vi "getTraceScreen.vi"(8 "error in":errorcluster, 11 "VISA in":refnum<visa-resource-name>="TCPIP0::172.16.1.100::inst0::INSTR") -> (0 "error out":errorcluster, 3 "VISA out":refnum<visa-resource-name>)   [LabVIEW 2023, in "Keysight.lvlib"]
uses:
  Keysight.lvlib
panel:
  out "*OPC?":string
  in  "FileName":string="FileName"
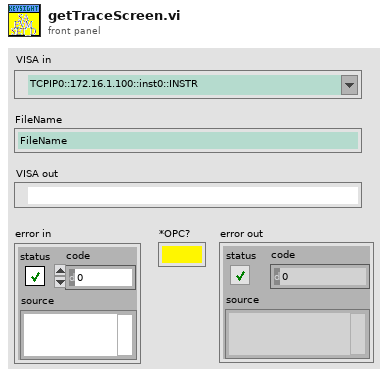
[diagram p1: front panel]
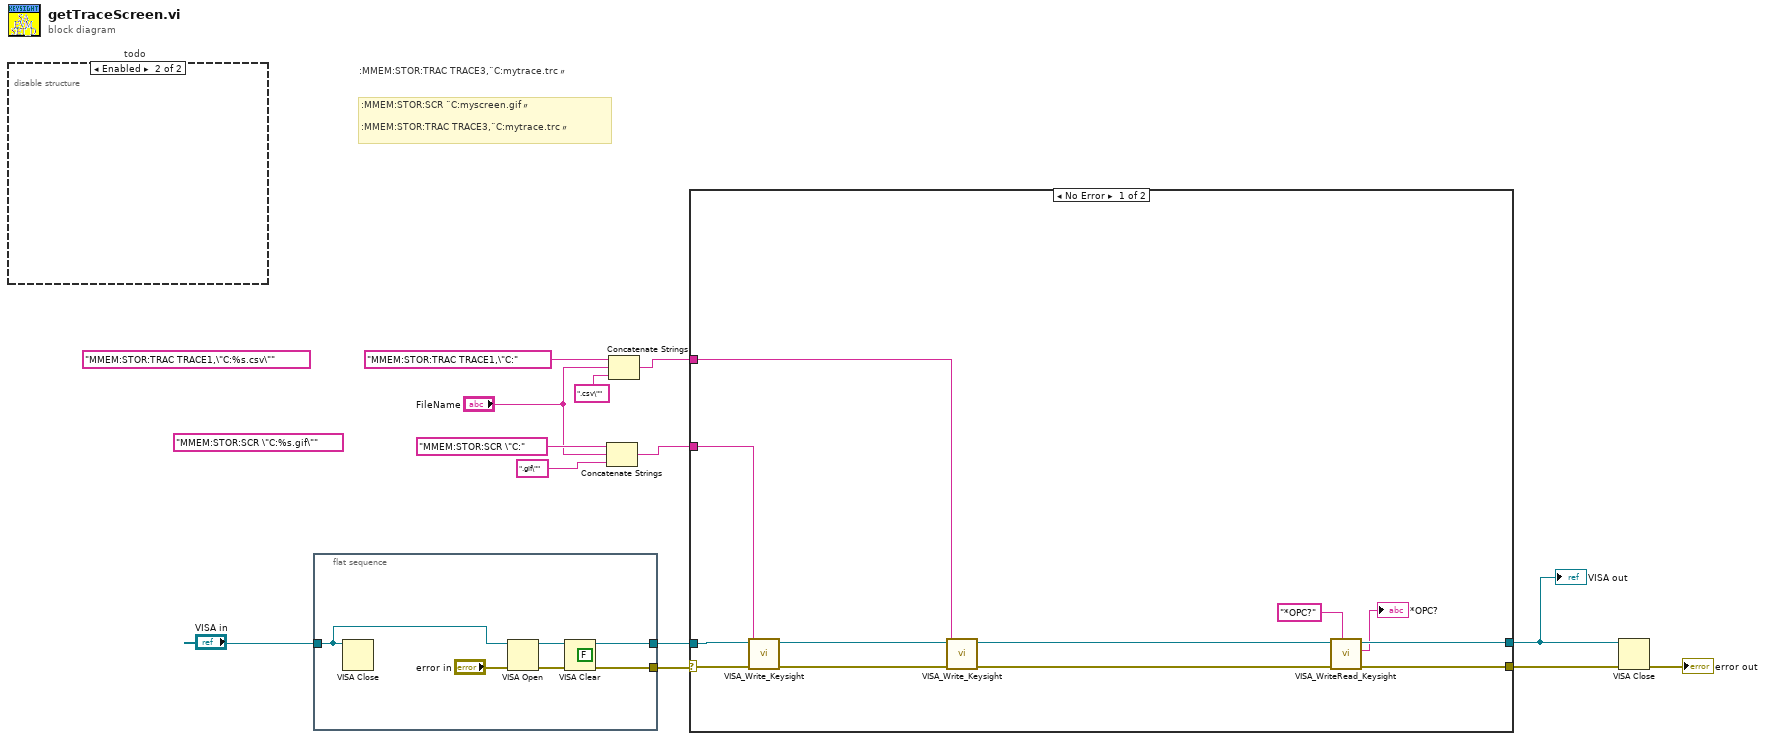
[diagram p0: block diagram]
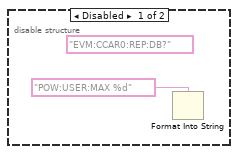
[diagram p2: hidden frame]
diagram:
  (unwired) "MMEM:STOR:TRAC TRACE1,\"C:%s.csv\"" ("write buffer")
  (unwired) "MMEM:STOR:SCR \"C:%s.gif\"" ("write buffer")
  # ":MMEM:STOR:SCR ¨C:myscreen.gif〃\n\n:MMEM:STOR:TRAC TRACE3,¨C:mytrace.trc〃"
  # ":MMEM:STOR:TRAC TRACE3,¨C:mytrace.trc〃"
  n1 = disable-structure "todo" shown="Enabled" {
    frame Disabled {
      (unwired) "EVM:CCAR0:REP:DB?" ("write buffer")
      n2 = Format Into String(format string="POW:USER:MAX %d") -> ()  [unwired: 3 in, 2 out]
    }
    frame Enabled {
    }
  }
  n3 = flat-sequence {
    tunnel: [w18] -> w6
    tunnel: [w17] -> w5
    tunnel: "VISA in" -> [w16]
    frame #0 {
      (unwired) FALSE ("duplicate session (F)")
      n4 = VISA Close(VISA resource name=w16) -> ()  [unwired: 1 in, 1 out]
      n5 = VISA Open(error in (no error)="error in", VISA resource name=w16) -> (VISA resource name=w19:refnum<visa-resource-name>, error out=w20:errorcluster)  [unwired: 3 in]
      n6 = VISA Clear(VISA resource name=w19, error in (no error)=w20) -> (VISA resource name out=w17:refnum<visa-resource-name>, error out=w18:errorcluster)
    }
  }
  n7 = Concatenate Strings("MMEM:STOR:SCR \"C:" ("write buffer"), "FileName", ".gif\"" ("string")) -> (w12:string)
  n8 = Concatenate Strings("MMEM:STOR:TRAC TRACE1,\"C:" ("write buffer"), "FileName", ".csv\"" ("string")) -> (w7:string)
  n9 = case shown="No Error" w6 {
    selector: w6 -> [w32 w34]
    tunnel: w12 -> [w31 _]
    tunnel: [w30 w34] -> w2
    tunnel: [w29 w33] -> w3
    tunnel: w7 -> [w24 _]
    tunnel: w5 -> [w21 w33]
    frame No Error {
      n10 = call "VISA_Write_Keysight.vi"("VISA CMD"=w31, "error in"=w32, "VISA in"=w21) -> ("error out"=w28:errorcluster, "VISA out"=w27:refnum<visa-resource-name>)  [unwired: 7 in]
      n11 = call "VISA_Write_Keysight.vi"("VISA CMD"=w24, "error in"=w28, "VISA in"=w27) -> ("error out"=w25:errorcluster, "VISA out"=w26:refnum<visa-resource-name>)  [unwired: 7 in]
      n12 = call "VISA_WriteRead_Keysight.vi"("VISA_CMD"="*OPC?", "error in"=w25, "VISA in"=w26) -> ("error out"=w30:errorcluster, "Response"=→"*OPC?":string, "VISA out"=w29:refnum<visa-resource-name>)  [unwired: 6 in]
    }
    frame Error {
    }
  }
  "VISA out" <- w3
  n13 = VISA Close(VISA resource name=w3, error in (no error)=w2) -> (error out=→"error out":errorcluster)
